vi "FlyWheel.vi"(1 "flyWheel Intake":dbl, 2 "flyDrive movement":dbl=0.5 format="%#_13g", 3 "Enum":enum16{"Drive", "Wheel", "Open"}(ring)) -> ()   [LabVIEW 2018]
uses:
  <vilib>/Rock Robotics/SystemInterfaces/DIO/FPGA_DIOPWMChannel.ctl
  <vilib>/Rock Robotics/SystemInterfaces/DIO/FPGA_DIOChannel.ctl
  <vilib>/Rock Robotics/WPI/Counter/WPI_CounterDigitalInputToDigitalSource.vi
  <vilib>/Rock Robotics/WPI/MotorControl/WPI_MotorControlOpen VictorSP.vi
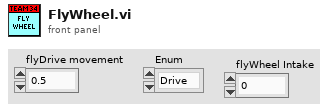
[diagram p1: front panel]
types:
  T1 = typedef "FPGA_DIOPWMChannel.ctl" = enum8{"PWM 0", "PWM 1", "PWM 2", "PWM 3", "PWM 4", "PWM 5", "PWM 6", "PWM 7", "PWM 8", "PWM 9", "PWM MXP 0", "PWM MXP 1", "PWM MXP 2", "PWM MXP 3", "PWM MXP 4", "PWM MXP 5", "PWM MXP 6", "PWM MXP 7", "PWM MXP 8", "PWM MXP 9", "Invalid"}
  T2 = typedef "FPGA_DIOChannel.ctl" = enum8{"DIO 0", "DIO 1", "DIO 2", "DIO 3", "DIO 4", "DIO 5", "DIO 6", "DIO 7", "DIO 8", "DIO 9", "DIO MXP 0", "DIO MXP 1", "DIO MXP 2", "DIO MXP 3", "DIO MXP 4", "DIO MXP 5", "DIO MXP 6", "DIO MXP 7", "DIO MXP 8", "DIO MXP 9", "DIO MXP 10", "DIO MXP 11", "DIO MXP 12", "DIO MXP 13", "DIO MXP 14", "DIO MXP 15", "SPI Port CS1", "SPI Port CS2", "SPI Port CS3", "SPI Port MISO", "SPI Port MOSI", "Invalid"}
  T3 = typedef "WPI_MotorControlDeviceRef.ctl" = cluster{"DeviceStatus":errorcluster, "Type":T4, "PWM":cluster{"PWM Channel":T1, "DeadBand":T5}, "CAN":cluster{"Device Number":u8, "SetOutput VI Ref":variant, "GetOutput VI Ref":variant, "Enable VI Ref":variant, "Disable VI Ref":variant, "Data":variant}, "Invert":bool, "DIO PWM":cluster{"PWM \"Enable\" Channel":T1, "DIOChannel":T2, "PWM Rate":dbl}}
  T4 = typedef "WPI_MotorControlType.ctl" = enum16{"PWM", "CAN", "DIO PWM"}
  T5 = typedef "WPI_PWMDeadband.ctl" = cluster{"Name":string, "maxPositivePwm":i32, "minPositivePwm":i32, "centerPwm":i32, "maxNegativePwm":i32, "minNegativePwm":i32, "angularRange":u16}
  T6 = typedef "WPI_DigitalInputDevRef.ctl" = cluster{"DevStatus":errorcluster, "DIO Channel":T2}
  T7 = typedef "FPGA_CounterEncoderSourceConvertionLVSourceType.ctl" = cluster{"DevStatus":errorcluster, "AnalogTriggerMode?":bool, "DigitalMode":cluster{"DIO Channel":T8}, "AnalogTriggerMode":cluster{"AnalogTriggerIndex":T9, "OutputType":T10}}
  T8 = typedef "FPGA_DIODigitalSourceChannel.ctl" = enum8{"DIO 0", "DIO 1", "DIO 2", "DIO 3", "DIO 4", "DIO 5", "DIO 6", "DIO 7", "DIO 8", "DIO 9", "DIO MXP 0", "DIO MXP 1", "DIO MXP 2", "DIO MXP 3", "DIO MXP 4", "DIO MXP 5", "DIO MXP 6", "DIO MXP 7", "DIO MXP 8", "DIO MXP 9", "DIO MXP 10", "DIO MXP 11", "DIO MXP 12", "DIO MXP 13", "DIO MXP 14", "DIO MXP 15", "SPI Port CS1", "SPI Port CS2", "SPI Port CS3", "SPI Port MISO", "SPI Port MOSI", "Disabled"}
  T9 = typedef "FPGA_AnalogTriggerIndex.ctl" = enum8{"Trig 0", "Trig 1", "Trig 2", "Trig 3", "Trig 4", "Trig 5", "Trig 6", "Trig 7", "Invalid"}
  T10 = typedef "FPGA_AnalogTriggerOutType.ctl" = enum16{"InWindow", "TriggerState", "Rising", "Falling"}
  T11 = typedef "WPI_EncoderDevRef.ctl" = cluster{"DevStatus":errorcluster, "EncoderIndex":T12, "CounterIndex":T13, "DistancePerCount":dbl, "Decoding Type":T14}
  T12 = typedef "FPGA_EncoderIdx.ctl" = enum8{"Enc 0", "Enc 1", "Enc 2", "Enc 3", "Enc 4", "Enc 5", "Enc 6", "Enc 7", "Invalid"}
  T13 = typedef "FPGA_CounterCtrSystemIndex.ctl" = enum8{"Ctr 0", "Ctr 1", "Ctr 2", "Ctr 3", "Ctr 4", "Ctr 5", "Ctr 6", "Ctr 7", "Invalid"}
  T14 = typedef "WPI_EncoderType.ctl" = enum16{"1x", "2x", "4x"}
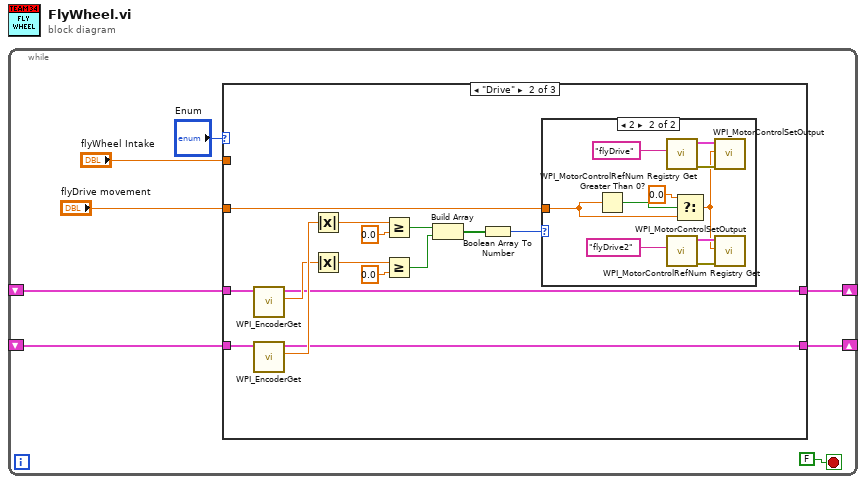
[diagram p0: block diagram]
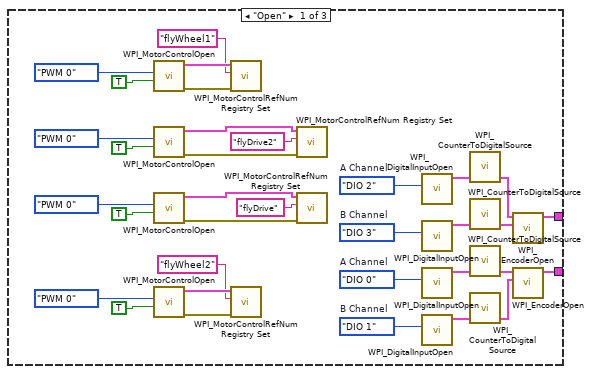
[diagram p2: hidden frame]
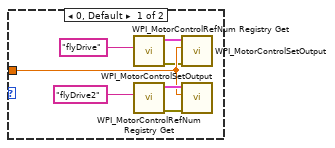
[diagram p3: hidden frame]
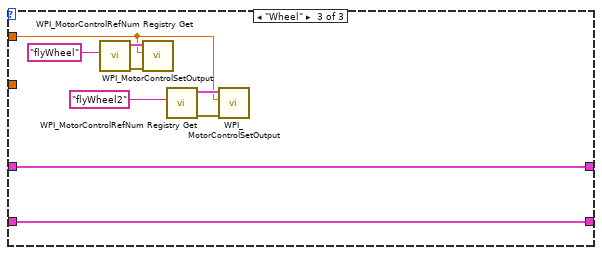
[diagram p4: hidden frame]
diagram:
  n1 = while {
    shift-right: [w5] -> _
    shift-left: _ -> [w2]
    shift-right: [w4] -> _
    shift-left: _ -> [w3]
    stop <- FALSE stop-if-true
    n2 = case shown="\"Drive\"" "Enum" {
      tunnel: "flyDrive movement" -> [_ w45 _]
      tunnel: [w14 w43 w79] -> w5
      tunnel: [w13 w44 w78] -> w4
      tunnel: w3 -> [_ w57 w78]
      tunnel: w2 -> [_ w56 w79]
      tunnel: "flyWheel Intake" -> [_ _ w75]
      frame "Open" {
        w15 = FPGA_DIOChannel."DIO 3"  # B Channel
        w16 = FPGA_DIOChannel."DIO 2"  # A Channel
        w26 = FPGA_DIOChannel."DIO 1"  # B Channel
        w25 = FPGA_DIOChannel."DIO 0"  # A Channel
        n3 = call-poly <vilib>:"WPI_MotorControlOpen.vi"("Eliminate Deadband"=TRUE, "PWM Channel"=FPGA_DIOPWMChannel."PWM 0") -> ("error out"=w39:errorcluster, "MotorControlDeviceRef"=w38:T3)  [unwired: 8 in]
        n4 = call-poly <vilib>:"WPI_MotorControlOpen.vi"("Eliminate Deadband"=TRUE, "PWM Channel"=FPGA_DIOPWMChannel."PWM 0") -> ("error out"=w36:errorcluster, "MotorControlDeviceRef"=w35:T3)  [unwired: 8 in]
        n5 = call-poly <vilib>:"WPI_MotorControlOpen.vi"("Eliminate Deadband"=TRUE, "PWM Channel"=FPGA_DIOPWMChannel."PWM 0") -> ("error out"=w33:errorcluster, "MotorControlDeviceRef"=w32:T3)  [unwired: 8 in]
        n6 = call-poly <vilib>:"WPI_MotorControlOpen.vi"("Eliminate Deadband"=TRUE, "PWM Channel"=FPGA_DIOPWMChannel."PWM 0") -> ("error out"=w42:errorcluster, "MotorControlDeviceRef"=w41:T3)  [unwired: 8 in]
        n7 = call <vilib>:"WPI_MotorControlRefNum Registry Set.vi"("error in (no error)"=w39, "refnum name"="flyWheel1", "MotorControlDevRef"=w38) -> ()  [unwired: 7 in, 2 out]
        n8 = call <vilib>:"WPI_MotorControlRefNum Registry Set.vi"("error in (no error)"=w42, "refnum name"="flyWheel2", "MotorControlDevRef"=w41) -> ()  [unwired: 7 in, 2 out]
        n9 = call <vilib>:"WPI_MotorControlRefNum Registry Set.vi"("error in (no error)"=w36, "refnum name"="flyDrive2", "MotorControlDevRef"=w35) -> ()  [unwired: 7 in, 2 out]
        n10 = call <vilib>:"WPI_MotorControlRefNum Registry Set.vi"("error in (no error)"=w33, "refnum name"="flyDrive", "MotorControlDevRef"=w32) -> ()  [unwired: 7 in, 2 out]
        n11 = call <vilib>:"WPI_DigitalInputOpen.vi"("DIO Channel"=w16) -> ("DigitalInputDevRef"=w19:T6)  [unwired: 1 in, 9 out]
        n12 = call <vilib>:"WPI_DigitalInputOpen.vi"("DIO Channel"=w15) -> ("DigitalInputDevRef"=w18:T6)  [unwired: 1 in, 9 out]
        n13 = call <vilib>:"WPI_DigitalInputOpen.vi"("DIO Channel"=w25) -> ("DigitalInputDevRef"=w22:T6)  [unwired: 1 in, 9 out]
        n14 = call <vilib>:"WPI_DigitalInputOpen.vi"("DIO Channel"=w26) -> ("DigitalInputDevRef"=w23:T6)  [unwired: 1 in, 9 out]
        n15 = call-poly <vilib>:"WPI_CounterToDigitalSource.vi"("DigitalInputDevRef"=w19) -> ("Digital Source"=w20:T7)  [unwired: 6 out]
        n16 = call-poly <vilib>:"WPI_CounterToDigitalSource.vi"("DigitalInputDevRef"=w18) -> ("Digital Source"=w17:T7)  [unwired: 6 out]
        n17 = call-poly <vilib>:"WPI_CounterToDigitalSource.vi"("DigitalInputDevRef"=w22) -> ("Digital Source"=w21:T7)  [unwired: 6 out]
        n18 = call-poly <vilib>:"WPI_CounterToDigitalSource.vi"("DigitalInputDevRef"=w23) -> ("Digital Source"=w24:T7)  [unwired: 6 out]
        n19 = call <vilib>:"WPI_EncoderOpen.vi"("BSource"=w17, "ASource"=w20) -> ("EncoderDevRef"=w14:T11)  [unwired: 6 in, 3 out]
        n20 = call <vilib>:"WPI_EncoderOpen.vi"("BSource"=w24, "ASource"=w21) -> ("EncoderDevRef"=w13:T11)  [unwired: 6 in, 3 out]
      }
      frame "Drive" {
        n21 = call <vilib>:"WPI_EncoderGet.vi"("EncoderDevRef"=w56) -> ("Distance"=w54:dbl, "EncoderDevRef"=w43:T11)  [unwired: 5 in, 4 out]
        n22 = call <vilib>:"WPI_EncoderGet.vi"("EncoderDevRef"=w57) -> ("Distance"=w55:dbl, "EncoderDevRef"=w44:T11)  [unwired: 5 in, 4 out]
        n23 = Absolute Value(x=w55) -> (abs(x)=w53:dbl)
        n24 = Absolute Value(x=w54) -> (abs(x)=w50:dbl)
        n25 = Greater Or Equal?(x=w53, y=0.0) -> (x >= y?=w49:bool)
        n26 = Greater Or Equal?(x=w50, y=0.0) -> (x >= y?=w48:bool)
        n27 = Build Array(w49, w48) -> (w47:bool[])
        n28 = Boolean Array To Number(Boolean array=w47) -> (number=w46:u32)
        n29 = case shown="2" w46 {
          tunnel: w45 -> [w62 w72]
          frame 0, Default {
            n30 = call <vilib>:"WPI_MotorControlRefNum Registry Get.vi"("refnum name"="flyDrive") -> ("error out"=w61:errorcluster, "MotorControlDevRef"=w64:T3)  [unwired: 9 in]
            n31 = call <vilib>:"WPI_MotorControlRefNum Registry Get.vi"("refnum name"="flyDrive2") -> ("error out"=w60:errorcluster, "MotorControlDevRef"=w63:T3)  [unwired: 9 in]
            n32 = call <vilib>:"WPI_MotorControlSetOutput.vi"("error in (no error)"=w61, "Output"=w62, "MotorControlDevRef"=w64) -> ()  [unwired: 6 in, 3 out]
            n33 = call <vilib>:"WPI_MotorControlSetOutput.vi"("error in (no error)"=w60, "Output"=w62, "MotorControlDevRef"=w63) -> ()  [unwired: 6 in, 3 out]
          }
          frame 2 {
            n34 = Greater Than 0?(x=w72) -> (x > 0?=w74:bool)
            n35 = call <vilib>:"WPI_MotorControlRefNum Registry Get.vi"("refnum name"="flyDrive") -> ("error out"=w70:errorcluster, "MotorControlDevRef"=w71:T3)  [unwired: 9 in]
            n36 = call <vilib>:"WPI_MotorControlRefNum Registry Get.vi"("refnum name"="flyDrive2") -> ("error out"=w67:errorcluster, "MotorControlDevRef"=w68:T3)  [unwired: 9 in]
            n37 = Select(t=0.0, s=w74, f=w72) -> (s? t:f=w65:dbl)
            n38 = call <vilib>:"WPI_MotorControlSetOutput.vi"("error in (no error)"=w70, "Output"=w65, "MotorControlDevRef"=w71) -> ()  [unwired: 6 in, 3 out]
            n39 = call <vilib>:"WPI_MotorControlSetOutput.vi"("error in (no error)"=w67, "Output"=w65, "MotorControlDevRef"=w68) -> ()  [unwired: 6 in, 3 out]
          }
        }
      }
      frame "Wheel" {
        n40 = call <vilib>:"WPI_MotorControlRefNum Registry Get.vi"("refnum name"="flyWheel") -> ("error out"=w77:errorcluster, "MotorControlDevRef"=w80:T3)  [unwired: 9 in]
        n41 = call <vilib>:"WPI_MotorControlSetOutput.vi"("error in (no error)"=w77, "Output"=w75, "MotorControlDevRef"=w80) -> ()  [unwired: 6 in, 3 out]
        n42 = call <vilib>:"WPI_MotorControlRefNum Registry Get.vi"("refnum name"="flyWheel2") -> ("error out"=w76:errorcluster, "MotorControlDevRef"=w81:T3)  [unwired: 9 in]
        n43 = call <vilib>:"WPI_MotorControlSetOutput.vi"("error in (no error)"=w76, "Output"=w75, "MotorControlDevRef"=w81) -> ()  [unwired: 6 in, 3 out]
      }
    }
  }
